vi "current_timestep.vi"() -> ()   [LabVIEW 2019]
panel:
  out "current timestep":dbl
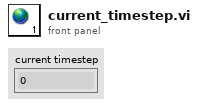
[diagram p1: front panel]
diagram:
